vi "Get Device Index.vi"(11 "LCD in":u32 format="%.0b") -> (3 "device index":i8)   [LabVIEW 2015, in "HD44780 FPGA.lvlib"]
uses:
  <vilib>/EmbeddedDisplay/Hitachi HD44780/FPGA/HD44780 FPGA.lvlib
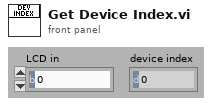
[diagram p1: front panel]
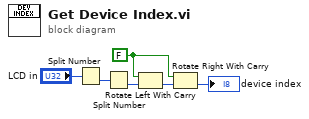
[diagram p0: block diagram]
diagram:
  w2 = FALSE ("carry")
  n1 = Split Number(x="LCD in") -> (lo(x)=w5:u16)  [unwired: 1 out]
  n2 = Split Number(x=w5) -> (lo(x)=w4:u8)  [unwired: 1 out]
  n3 = Rotate Left With Carry(2:w4, 3:w2) -> (0:w3:u8)  [unwired: 1 out]
  n4 = Rotate Right With Carry(2:w3, 3:w2) -> (0:→"device index":u8)  [unwired: 1 out]
